vi "UDP Date Time and Match Status to RPI.vi"(6 "Address":u32, 9 "Port":u16, 10 "port":refnum<k16>) -> ()   [LabVIEW 2025]
uses:
  <vilib>/Rock Robotics/SystemInterfaces/NetworkCommunication/NetComm_MatchType.ctl
  <vilib>/Rock Robotics/WPI/DriverStation/WPI_DriverStationRobotMode2.ctl
panel:
  out "Match Type":T1
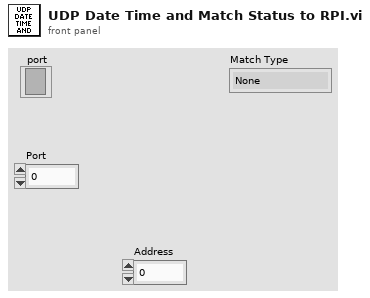
[diagram p1: front panel]
types:
  T1 = typedef "NetComm_MatchType.ctl" = enum32{"None", "Practice", "Qualification", "Elimination"}
  T2 = typedef "WPI_DriverStationRobotMode2.ctl" = enum16{"Autonomous Disabled", "Autonomous Enabled", "Teleop Disabled", "Teleop Enabled", "Disconnected", "Finish", "Test Disabled", "Test Enabled", "Emergency Stopped"}
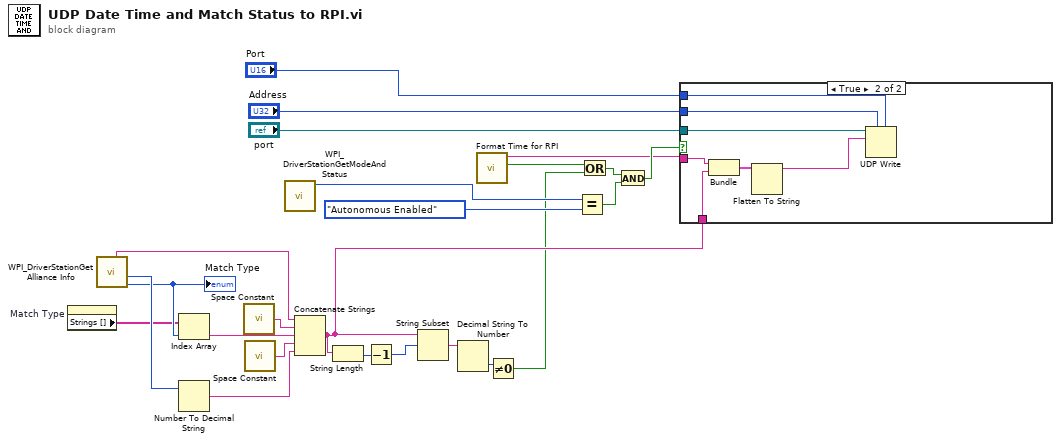
[diagram p0: block diagram]
diagram:
  n1 = property on="Match Type" class="Enum (strict)"() -> ("Strings []"=w7:string[])  [unwired: 2 in, 2 out]
  n2 = call <vilib>:"WPI_DriverStationGet Alliance Info.vi"() -> ("Match Type"=w15:T1, "Match Number"=w17:u16, "Event Name"=w12:string)  [unwired: 6 in, 3 out]
  "Match Type" <- w15
  n3 = Index Array(array=w7, index=w15) -> (element=w16:string)
  n4 = Number To Decimal String(number=w17) -> (decimal integer string=w18:string)  [unwired: 1 in]
  n5 = call <vilib>:"Space Constant.vi"() -> ("String"=w13:string)
  n6 = call <vilib>:"Space Constant.vi"() -> ("String"=w14:string)
  n7 = call <vilib>:"WPI_DriverStationGetModeAndStatus.vi"() -> ("Robot Mode"=w21:T2)  [unwired: 10 in, 1 out]
  n8 = Concatenate Strings(w12, w13, w16, w14, w18) -> (w5:string)
  n9 = String Length(string=w5) -> (length=w6:i32)
  n10 = Decrement(x=w6) -> (x-1=w4:i32)
  n11 = String Subset(string=w5, offset (0)=w4) -> (substring=w3:string)  [unwired: 1 in]
  n12 = Decimal String To Number(string=w3) -> (number=w2:i32)  [unwired: 2 in, 1 out]
  n13 = call "Format Time for RPI.vi"() -> ("is date valid?"=w20:bool, "date/time string"=w11:string)  [unwired: 10 in]
  n14 = Not Equal To 0?(x=w2) -> (x != 0?=w1:bool)
  n15 = Equal?(x=w21, y=WPI_DriverStationRobotMode2."Autonomous Enabled") -> (x = y?=w23:bool)
  n16 = Or(x=w20, y=w1) -> (x .or. y?=w19:bool)
  n17 = And(x=w19, y=w23) -> (x .and. y?=w24:bool)
  n18 = case shown="True" w24 {
    tunnel: "Address" -> [_ w31]
    tunnel: "Port" -> [_ w30]
    tunnel: "port" -> [_ w29]
    tunnel: w11 -> [_ w26]
    tunnel: w5 -> [_ w28]
    frame False {
    }
    frame True {
      n19 = Bundle("date/time string"=w26, w28) -> (w27:cluster{"date/time string":string, string})  [unwired: 1 in]
      n20 = Flatten To String(anything=w27) -> (data string=w25:string)  [unwired: 3 in, 2 out]
      n21 = UDP Write(address=w31, port or service name=w30, connection ID=w29, data in=w25) -> ()  [unwired: 2 in, 2 out]
    }
  }
